vi "CreateQueue.xio.vi"(2 "错误输入（无错误）":errorcluster, 3 "名称":string) -> (0 "错误输出":errorcluster)   [LabVIEW 2014]
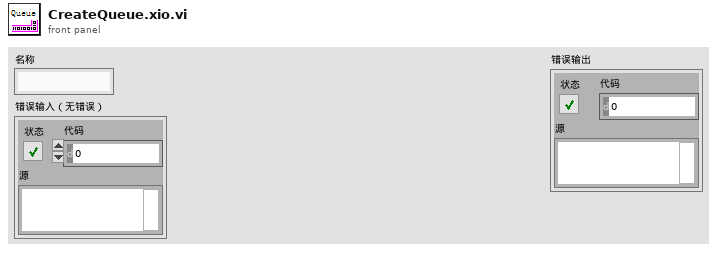
[diagram p1: front panel]
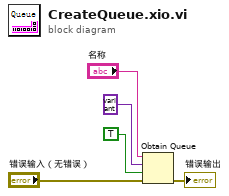
[diagram p0: block diagram]
diagram:
  n1 = Obtain Queue(name (unnamed)="名称", element data type=variant ("元素数据类型"), create if not found? (T)=TRUE ("如未找到则创建？(T)"), error in (no error)="错误输入（无错误）") -> (error out=→"错误输出":errorcluster)  [unwired: 1 in, 2 out]
